vi "Load Maze Gen.vi"(8 "error in (no error)":errorcluster, 11 "Maze Level":string) -> (0 "error out":errorcluster, 3 "MazeGen":refnum<class "MazeGen.lvclass">)   [LabVIEW 2020, in "Maze.lvlib" / "MazeGen.lvclass"]
doc: "Loads the PPL that contains the logic for generating the specific maze level. <b>Basic</b> is built into the MazeGen class but other algorithms are loaded dynamically from disk to support being distributed after the start of the challenge.\n\n<b>Errors</b>\n\n<b>-124100</b> is thrown if the specific algorithm (PPL) was not found or able to be loaded."
uses:
  MazeGen.lvclass
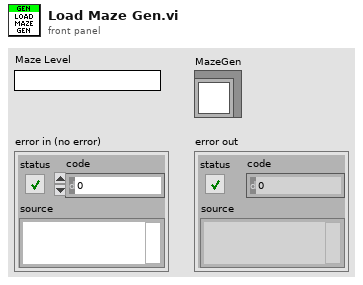
[diagram p1: front panel]
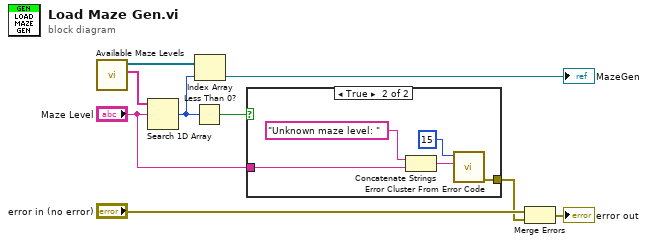
[diagram p0: block diagram]
diagram:
  n1 = call "Available Maze Levels.vi"() -> ("Names"=w7:string[], "Available Mazes"=w6:refnum<class "MazeGen.lvclass">[])  [unwired: 10 in]
  n2 = Search 1D Array(1D array=w7, element="Maze Level") -> (index of element=w4:i32)  [unwired: 1 in]
  n3 = Less Than 0?(x=w4) -> (x < 0?=w3:bool)
  n4 = Index Array(array=w6, index=w4) -> (element=→"MazeGen":refnum<class "MazeGen.lvclass">)
  n5 = case shown="True" w3 {
    tunnel: "Maze Level" -> [_ w11]
    tunnel: [_ w10] -> w1
    frame False {
    }
    frame True {
      n6 = Concatenate Strings("Unknown maze level: ", w11) -> (w13:string)
      n7 = call <vilib>:"Error Cluster From Error Code.vi"("error message (\"\")"=w13, "error code (0)"=15) -> ("error out"=w10:errorcluster)  [unwired: 7 in]
    }
  }
  n8 = Merge Errors("error in (no error)", w1) -> (→"error out":errorcluster)
